vi "Flag_Clear.vi"(8 "error in (no error)":errorcluster) -> (0 "error out":errorcluster)   [LabVIEW 2016, in "SeqProcessor.lvlib"]
uses:
  SeqProcessor.lvlib
  controls/Flag.ctl
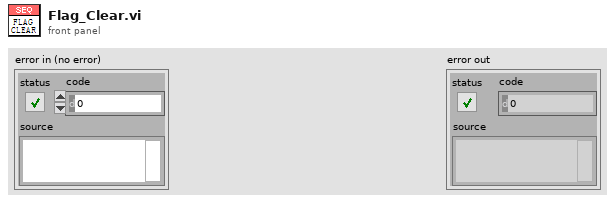
[diagram p1: front panel]
types:
  T1 = typedef "SeqProcessor.lvlib/Flag.ctl" = cluster{"SingleStep":bool, "Pause":bool, "Stop":bool, "StepbyStep":bool}
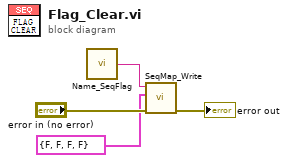
[diagram p0: block diagram]
diagram:
  n1 = call "Name_SeqFlag.vi"() -> ("SeqFlag"=w2:string)  [unwired: 5 in]
  n2 = call "SeqMap_Write.vi"("error in (no error)"="error in (no error)", "Value"=T1 {"SingleStep"=FALSE, "Pause"=FALSE, "Stop"=FALSE, "StepbyStep"=FALSE} ("Flag"), "Tag"=w2) -> ("error out"=→"error out":errorcluster)  [unwired: 8 in]
